vi "RSZVB Set Converter Port Assignment.vi"(8 "error in (no error)":errorcluster {"code" format="%.0x"}, 9 "Serial Number (\"\")":string, 10 "Port (1)":i32=1, 11 "VISA resource name":refnum<visa-resource-name>) -> (0 "error out":errorcluster {"code" format="%.0x"}, 3 "VISA resource name out":refnum<visa-resource-name>)   [LabVIEW 2011]
doc: "This VI assigns a R&S ZCxxx converter to port no. <Port>\n\nNote(s): \n\n(1) The adequate converter type and test setup have to be set beforehand using \nrszvb_SetFrequencyConversionType and \nrszvb_SetFrequencyConversionSource, respectively.\n\nRemote-control command(s):\n[SENSe<Ch>:]CONVerter:ASSign<Port>"
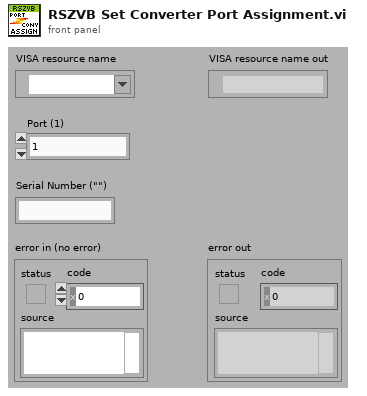
[diagram p1: front panel]
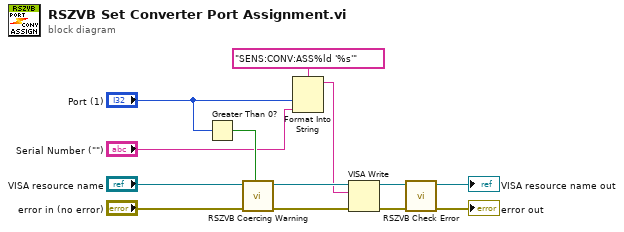
[diagram p0: block diagram]
diagram:
  n1 = Greater Than 0?(x="Port (1)") -> (x > 0?=w7:bool)
  n2 = call "RSZVB Coercing Warning.vi"("In Range?"=w7, "error in (no error)"="error in (no error)", "VISA session"="VISA resource name") -> ("error out"=w11:errorcluster, "dup VISA session"=w12:refnum<visa-resource-name>)  [unwired: 7 in]
  n3 = Format Into String(format string="SENS:CONV:ASS%ld '%s'", "Port (1)", "Serial Number (\"\")") -> (resulting string=w8:string)  [unwired: 2 in, 1 out]
  n4 = VISA Write(VISA resource name=w12, write buffer=w8, error in (no error)=w11) -> (VISA resource name out=w9:refnum<visa-resource-name>, error out=w10:errorcluster)  [unwired: 1 out]
  n5 = call "RSZVB Check Error.vi"("error in (no error)"=w10, "VISA session"=w9) -> ("error out"=→"error out":errorcluster, "dup VISA session"=→"VISA resource name out":refnum<visa-resource-name>)  [unwired: 8 in]
